vi "MD5 core.vi"(7 "Input String":string, 8 "s4":u32=271733878 format="%.0x", 9 "s3":u32=2562383102 format="%.0x", 10 "s2":u32=4023233417 format="%.0x", 11 "s1":u32=1732584193 format="%.0x") -> (0 "s4":u32, 1 "s3":u32, 2 "s2":u32, 3 "s1":u32)   [LabVIEW 2019, in "Tools.lvlib"]
doc: "This VI contains the core of the MD5 algorithm."
uses:
  Tools.lvlib
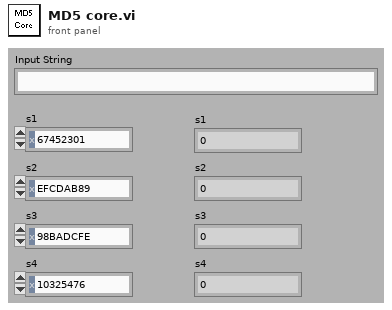
[diagram p1: front panel]
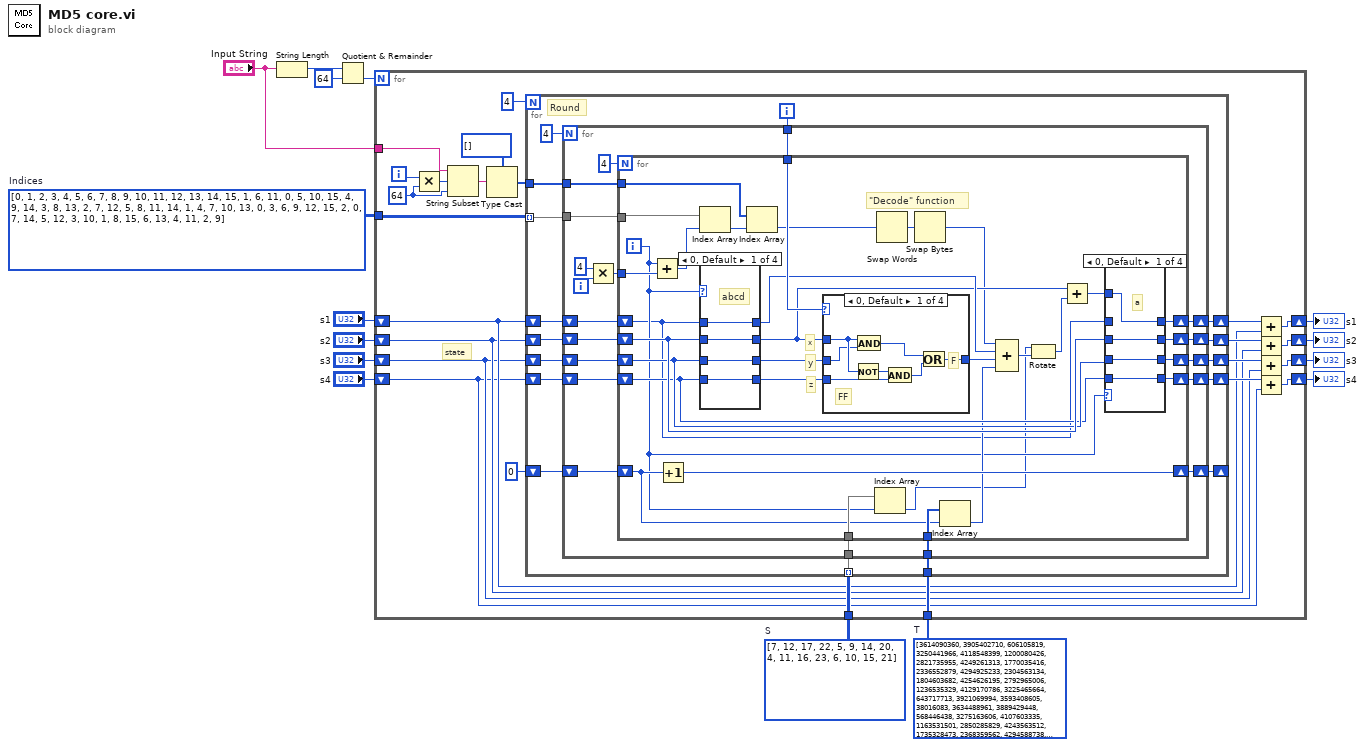
[diagram p0: block diagram]
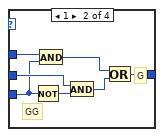
[diagram p2: hidden frame]
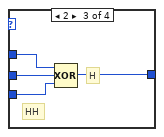
[diagram p3: hidden frame]
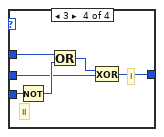
[diagram p4: hidden frame]
diagram:
  w9 = i32[][] [[7, 12, 17, 22], [5, 9, 14, 20], [4, 11, 16, 23], [6, 10, 15, 21]]  # S
  w10 = u32[] [3614090360, 3905402710, 606105819, 3250441966, 4118548399, 1200080426, 2821735955, 4249261313, 1770035416, 2336552879, 4294925233, 2304563134, 1804603682, 4254626195, 2792965006, 1236535329, 4129170786, 3225465664, 643717713, 3921069994, 3593408605, 38016083, 3634488961, 3889429448, 568446438, 3275163606, 4107603335, 1163531501, 2850285829, 4243563512, 1735328473, 2368359562, 4294588738, 2272392833, 1839030562, 4259657740, 2763975236, 1272893353, 4139469664, 3200236656, 681279174, 3936430074, 3572445317, 76029189, 3654602809, 3873151461, 530742520, 3299628645, 4096336452, 1126891415, 2878612391, 4237533241, 1700485571, 2399980690, 4293915773, 2240044497, 1873313359, 4264355552, 2734768916, 1309151649, 4149444226, 3174756917, 718787259, 3951481745]  # T
  w11 = i32[][] [[0, 1, 2, 3, 4, 5, 6, 7, 8, 9, 10, 11, 12, 13, 14, 15], [1, 6, 11, 0, 5, 10, 15, 4, 9, 14, 3, 8, 13, 2, 7, 12], [5, 8, 11, 14, 1, 4, 7, 10, 13, 0, 3, 6, 9, 12, 15, 2], [0, 7, 14, 5, 12, 3, 10, 1, 8, 15, 6, 13, 4, 11, 2, 9]]  # Indices
  n1 = String Length(string="Input String") -> (length=w14:i32)
  n2 = Quotient & Remainder(x=w14, y=64) -> (floor(x/y)=w15:i32)  [unwired: 1 out]
  n3 = for {
    N: w15 -> [_]
    tunnel: w11 -> [w33]
    tunnel: w10 -> [w32]
    tunnel: w9 -> [w31]
    shift-right: [w30] -> w8
    shift-left: "s1" -> [w26]
    shift-right: [w29] -> w7
    shift-left: "s2" -> [w25]
    shift-right: [w28] -> w6
    shift-left: "s3" -> [w24]
    shift-right: [w27] -> w5
    shift-left: "s4" -> [w23]
    tunnel: "Input String" -> [w21]
    i -> [w22]
    w16 = 64 ("y")
    # "state"
    n4 = Multiply(x=w22, y=w16) -> (x*y=w17:i32)
    n5 = String Subset(string=w21, offset (0)=w17, length (rest)=w16) -> (substring=w20:string)
    n6 = Type Cast(type=u32[] [], x=w20) -> (*(type *) &x=w18:u32[])
    n7 = for {
      N: 4 -> [_]
      shift-right: [w50] -> w36
      shift-left: w26 -> [w51]
      shift-right: [w49] -> w37
      shift-left: w25 -> [w52]
      shift-right: [w48] -> w38
      shift-left: w24 -> [w53]
      shift-right: [w47] -> w39
      shift-left: w23 -> [w54]
      tunnel: w33 -> [w46] mode=indexing
      tunnel: w31 -> [w45] mode=indexing
      tunnel: w18 -> [w44]
      shift-right: [w41] -> _
      shift-left: 0 -> [w42]
      tunnel: w32 -> [w40]
      i -> [w55]
      # "Round"
      n8 = for {
        N: 4 -> [_]
        tunnel: w55 -> [w74]
        shift-right: [w67] -> w47
        shift-left: w54 -> [w68]
        shift-right: [w66] -> w48
        shift-left: w53 -> [w69]
        shift-right: [w72] -> w49
        shift-left: w52 -> [w70]
        shift-right: [w73] -> w50
        shift-left: w51 -> [w71]
        tunnel: w46 -> [w65]
        tunnel: w45 -> [w64]
        tunnel: w44 -> [w60]
        shift-right: [w57] -> w41
        shift-left: w42 -> [w58]
        tunnel: w40 -> [w56]
        i -> [w63]
        n9 = Multiply(x=4, y=w63) -> (x*y=w61:i32)
        n10 = for {
          N: 4 -> [_]
          tunnel: w74 -> [w88]
          shift-right: [w98] -> w67
          shift-left: w68 -> [w93]
          shift-right: [w97] -> w66
          shift-left: w69 -> [w94]
          shift-right: [w96] -> w72
          shift-left: w70 -> [w95]
          shift-right: [w99] -> w73
          shift-left: w71 -> [w76]
          tunnel: w65 -> [w106]
          tunnel: w64 -> [w105]
          tunnel: w61 -> [w92]
          tunnel: w60 -> [w102]
          shift-right: [w89] -> w57
          shift-left: w58 -> [w90]
          tunnel: w56 -> [w91]
          i -> [w80]
          # "\"Decode\" function"
          # "z"
          # "y"
          # "x"
          n11 = Add(x=w80, y=w92) -> (x+y=w104:i32)
          n12 = Increment(x=w90) -> (x+1=w89:i32)
          n13 = Index Array(array=w106, index=w104) -> (element=w103:i32)
          n14 = case shown="0, Default" w80 {
            tunnel: w76 -> [w150 w153 w156 w160]
            tunnel: w95 -> [w149 w152 w155 w162]
            tunnel: w94 -> [w148 w151 w158 w161]
            tunnel: w93 -> [w147 w154 w157 w159]
            tunnel: [w150 w154 w158 w162] -> w83
            tunnel: [w149 w153 w157 w161] -> w82
            tunnel: [w148 w152 w156 w159] -> w101
            tunnel: [w147 w151 w155 w160] -> w100
            frame 0, Default {
              # "abcd"
            }
            frame 1 {
              # "dabc"
            }
            frame 2 {
              # "cdab"
            }
            frame 3 {
              # "bcda"
            }
          }
          n15 = Index Array(array=w102, index=w103) -> (element=w78:u32)
          n16 = case shown="0, Default" w88 {
            tunnel: w82 -> [w110 w116 w123 w127]
            tunnel: w101 -> [w109 w115 w124 w126]
            tunnel: w100 -> [w108 w114 w122 w125]
            tunnel: [w107 w117 w121 w128] -> w84
            frame 0, Default {
              # "FF"
              # "F"
              n17 = Not(x=w110) -> (.not. x?=w113:u32)
              n18 = And(x=w110, y=w109) -> (x .and. y?=w112:u32)
              n19 = And(x=w113, y=w108) -> (x .and. y?=w111:u32)
              n20 = Or(x=w112, y=w111) -> (x .or. y?=w107:u32)
            }
            frame 1 {
              # "GG"
              # "G"
              n21 = Not(x=w114) -> (.not. x?=w118:u32)
              n22 = And(x=w116, y=w114) -> (x .and. y?=w119:u32)
              n23 = And(x=w115, y=w118) -> (x .and. y?=w120:u32)
              n24 = Or(x=w119, y=w120) -> (x .or. y?=w117:u32)
            }
            frame 2 {
              # "H"
              # "HH"
              n25 = Compound Arithmetic op=XOR(w123, w124, w122) -> (w121:u32)
            }
            frame 3 {
              # "I"
              # "II"
              n26 = Not(x=w125) -> (.not. x?=w130:u32)
              n27 = Or(x=w127, y=w130) -> (x .or. y?=w129:u32)
              n28 = Exclusive Or(1:w126, 2:w129) -> (0:w128:u32)
            }
          }
          n29 = Index Array(array=w105, index=w80) -> (element=w75:i32)
          n30 = Swap Words(1:w78) -> (0:w79:u32)
          n31 = Swap Bytes(anything=w79) -> (byte swapped=w77:u32)
          n32 = Index Array(array=w91, index=w90) -> (element=w85:u32)
          n33 = Compound Arithmetic op=ADD(w77, w83, w84, w85) -> (w87:u32)
          n34 = Rotate(1:w87, 2:w75) -> (0:w81:u32)
          n35 = Add(x=w82, y=w81) -> (x+y=w86:u32)
          n36 = case shown="0, Default" w80 {
            tunnel: w86 -> [w134 w138 w142 w146]
            tunnel: [w134 w137 w141 w145] -> w99
            tunnel: [w131 w138 w139 w143] -> w98
            tunnel: [w132 w135 w142 w144] -> w97
            tunnel: [w133 w136 w140 w146] -> w96
            tunnel: w76 -> [_ w137 w141 w145]
            tunnel: w95 -> [w133 w136 w140 _]
            tunnel: w94 -> [w132 w135 _ w144]
            tunnel: w93 -> [w131 _ w139 w143]
            frame 0, Default {
              # "a"
            }
            frame 1 {
              # "d"
            }
            frame 2 {
              # "c"
            }
            frame 3 {
              # "b"
            }
          }
        }
      }
    }
    n37 = Add(x=w36, y=w26) -> (x+y=w30:u32)
    n38 = Add(x=w37, y=w25) -> (x+y=w29:u32)
    n39 = Add(x=w38, y=w24) -> (x+y=w28:u32)
    n40 = Add(x=w39, y=w23) -> (x+y=w27:u32)
  }
  "s1" <- w8
  "s2" <- w7
  "s3" <- w6
  "s4" <- w5
